vi "Create Archive.vi"() -> (0 "filename":string)   [LabVIEW 2013]
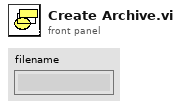
[diagram p1: front panel]
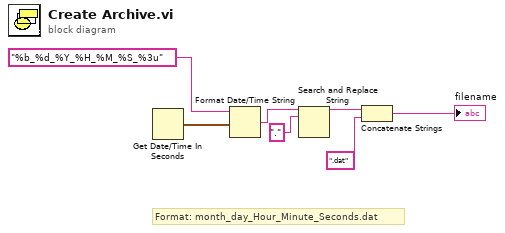
[diagram p0: block diagram]
diagram:
  # "Format: month_day_Hour_Minute_Seconds.dat"
  n1 = Get Date/Time In Seconds() -> (seconds since 1Jan1904=w7:timestamp)
  n2 = Format Date/Time String(time format string (%c)="%b_%d_%Y_%H_%M_%S_%3u", seconds (now)=w7) -> (date/time string=w5:string)  [unwired: 1 in]
  n3 = Search and Replace String(input string=w5, search string=".") -> (result string=w3:string)  [unwired: 6 in, 3 out]
  n4 = Concatenate Strings(w3, ".dat" ("string")) -> (→"filename":string)
